vi "Code 0.0.3.vi"() -> ()   [LabVIEW 2017]
uses:
  <vilib>/Instr/_visa.llb/VISA Open Access Mode.ctl
  <vilib>/Instr/_visa.llb/Select Event Type.ctl
  <vilib>/Utility/config.llb/Read Key (String).vi
  <vilib>/Utility/config.llb/Write Key (String).vi
  <vilib>/Instr/_visa.llb/VISA Configure Serial Port (Instr).vi
  <vilib>/Utility/config.llb/NI_LVConfig.lvlib
panel:
  in  "stop 7":bool
  in  "stop 6":bool
  out "Error List":string
  in  "Flash Baud":u32(ring)=115200 caption="Flash Baudrate" items=["4800"=4800, "9600"=9600, "19200"=19200, "38400"=38400, "57600"=57600, "115200"=115200, "230400"=230400, "460800"=460800, "921600"=921600]
  in  "cmd Baud":u32(ring)=230400 items=["4800"=4800, "9600"=9600, "19200"=19200, "38400"=38400, "57600"=57600, "115200"=115200, "230400"=230400, "460800"=460800, "921600"=921600]
  in  "COM Port":refnum<visa-resource-name>="COM4"
  in  "Next Button":bool
  in  "File Path Control":path
  out "COM Port":bool
  out "CheckSumArray":u16[][](array[numeric]) format="%.0x"
  out "CheckSum DataB":u16 format="%.0x"
  out "CheckSum Data":u16 format="%.0x"
  out "Array 3":u16[][](array[numeric]) format="%.0x"
  out "Num of Data packet":i32
  out "Size of Text File":i32
  out "Full Text File":u8[](array[numeric]) format="%.0x"
  out "All bytes in file in HEX U8":u8[](array[numeric]) format="%02x"
  out "sumHeader":u16 format="%.0x"
  out "error out":errorcluster
  # "Ver 1.0.5"
  # "© Redler Technologies. All Rights Reserved"
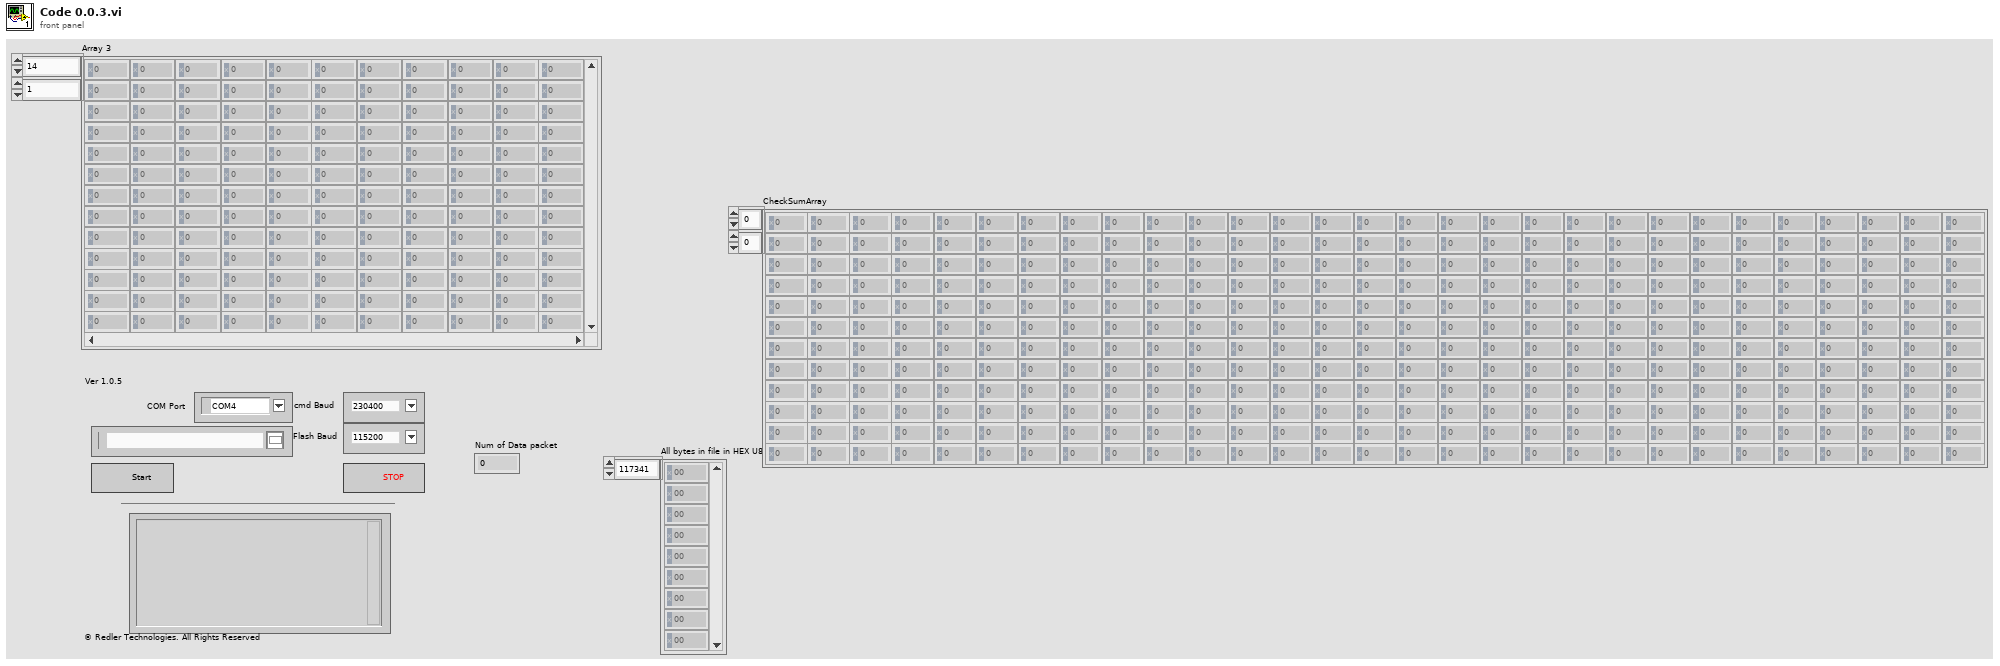
[diagram p1: front panel]
types:
  T1 = typedef "NI_LVConfig.lvlib/Config Data RefNum.ctl" = refnum<k1>
  T2 = typedef "VISA Open Access Mode.ctl" = u32
  T3 = typedef "Select Event Type.ctl" = u32
  T4 = enum16{"open", "replace", "create", "open or create", "replace or create", "replace or create with confirmation"}
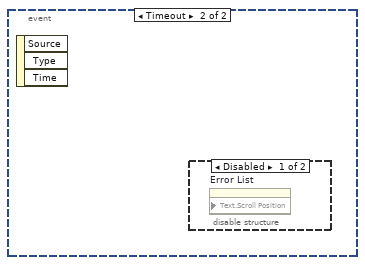
[diagram p3: hidden frame]
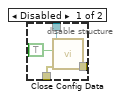
[diagram p5: hidden frame]
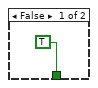
[diagram p6: hidden frame]
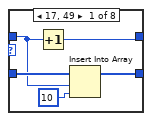
[diagram p7: hidden frame]
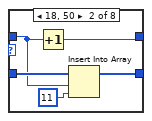
[diagram p8: hidden frame]
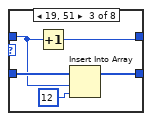
[diagram p9: hidden frame]
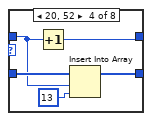
[diagram p10: hidden frame]
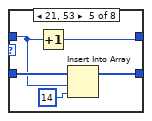
[diagram p11: hidden frame]
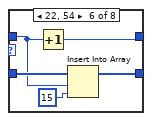
[diagram p12: hidden frame]
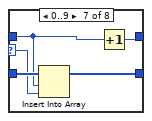
[diagram p13: hidden frame]
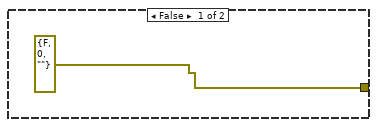
[diagram p15: hidden frame]
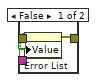
[diagram p16: hidden frame]
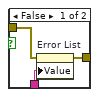
[diagram p18: hidden frame]
diagram:
  w8 = u32 230400 items=["4800"=4800, "9600"=9600, "19200"=19200, "38400"=38400, "57600"=57600, "115200"=115200, "230400"=230400, "460800"=460800, "921600"=921600] ("cmd Baud")
  w9 = u32 230400 items=["4800"=4800, "9600"=9600, "19200"=19200, "38400"=38400, "57600"=57600, "115200"=115200, "230400"=230400, "460800"=460800, "921600"=921600] ("Flash Baud")
  w18 = u32 230400 ("default (0 I32)")
  w3 = "Firmware Path" ("key")
  w4 = "Rayon" ("section")
  n1 = control-ref of="This VI"() -> (w40:refnum<vi>)
  n2 = invoke class="VI" method="Default Vals.Reinit All"(reference=w40, error in=errorcluster {"status"=FALSE, "code"=0, "source"=""} ("error in (no error)")) -> (error out=w7:errorcluster)  [unwired: 1 in, 2 out]
  n3 = property on="Flash Baud" class="Ring (strict)"(error in=w7, "Value"=w9) -> (error out=w10:errorcluster)  [unwired: 1 in, 1 out]
  n4 = property on="cmd Baud" class="Ring (strict)"(error in=w10, "Value"=w8) -> (error out=w6:errorcluster)  [unwired: 1 in, 1 out]
  n5 = call <vilib>:"Application Directory.vi"() -> ("Application Directory"=w38:path)
  n6 = Build Path(base path=w38, name or relative path="data\\RayonSerialProgramerConfigurationFile.ini") -> (appended path=w29:path)
  n7 = call <vilib>:"Open Config Data.vi"("error in (no error)"=w6, "create file if necessary (T)"=FALSE, "configuration file path"=w29) -> ("error out"=w34:errorcluster, "refnum"=w35:T1)  [unwired: 7 out]
  n8 = call-poly <vilib>:"Read Key.vi"("section"=w4, "error in (no error)"=w34, "key"=w3, "refnum"=w35) -> ("error out"=w1:errorcluster, "value"=w33:string, "refnum out"=w5:T1)  [unwired: 2 in, 3 out]
  n9 = String To Path(string=w33) -> (path=w32:path)
  n10 = property on="File Path Control" class="Path"(error in=w1, "Value"=w32) -> (error out=w2:errorcluster)  [unwired: 1 in, 1 out]
  n11 = call-poly <vilib>:"Read Key.vi"("section"=w4, "error in (no error)"=w2, "key"="COM", "refnum"=w5) -> ("error out"=w22:errorcluster, "value"=w14:string, "refnum out"=w27:T1)  [unwired: 2 in, 3 out]
  n12 = Type Cast(type=refnum<visa-resource-name> "COM1" ("UUT COM Port 2"), x=w14) -> (*(type *) &x=w13:refnum<visa-resource-name>)
  n13 = property on="COM Port" class="VISAName"("Value"=w13) -> ()  [unwired: 2 in, 2 out]
  n14 = call-poly <vilib>:"Read Key.vi"("section"=w4, "error in (no error)"=w22, "key"="Flash Baud", "refnum"=w27) -> ("error out"=w21:errorcluster, "value"=w20:string, "refnum out"=w28:T1)  [unwired: 2 in, 3 out]
  n15 = Decimal String To Number(string=w20, default (0L)=w18) -> (number=w16:u32)  [unwired: 1 in, 1 out]
  n16 = property on="Flash Baud" class="Ring (strict)"("Value"=w16) -> ()  [unwired: 2 in, 2 out]
  n17 = call-poly <vilib>:"Read Key.vi"("section"=w4, "error in (no error)"=w21, "key"="Boot Baud", "refnum"=w28) -> ("error out"=w11:errorcluster, "value"=w19:string, "refnum out"=w26:T1)  [unwired: 2 in, 3 out]
  n18 = Decimal String To Number(string=w19, default (0L)=w18) -> (number=w17:u32)  [unwired: 1 in, 1 out]
  n19 = property on="cmd Baud" class="Ring (strict)"("Value"=w17) -> ()  [unwired: 2 in, 2 out]
  n20 = call <vilib>:"Close Config Data.vi"("error in (no error)"=w11, "refnum"=w26) -> ("error out"=w12:errorcluster)  [unwired: 1 in, 8 out]
  n21 = while {
    tunnel: w12 -> [w45]
    tunnel: w4 -> [w107]
    tunnel: w3 -> [w106]
    tunnel: [w108] -> w31
    tunnel: w29 -> [w105]
    stop <- FALSE stop-if-true
    w96 = FALSE ("Next Button")
    w117 = T2 0 items=["VISA Defaults"=0, "Exclusive Lock"=1, "Load Configured Settings"=4] ("Access Mode")
    # "Convert from U8 to U16 to build a word (Header)"
    # "build U8 HEX values"
    # "Convert from U8 to U16 to build a word (Data)"
    # "Convert ASCII string to HEX values"
    n22 = property on="File Path Control" class="Path"(error in=w45, "PTooLngToFt"=enum32{"Abbreviate Path", "Clip Path"}."Abbreviate Path" ("Path Too Long To Fit")) -> ()  [unwired: 1 in, 2 out]
    n23 = property on="stop 6" class="Bool (strict)"(error in=w45, "Value"=FALSE ("stop 6")) -> (error out=w54:errorcluster)  [unwired: 1 in, 1 out]
    n24 = while {
      tunnel: ["COM Port"] -> w43
      tunnel: ["Flash Baud"] -> w119
      tunnel: ["cmd Baud"] -> w118
      tunnel: ["File Path Control"] -> w57
      tunnel: w107 -> [w1024]
      tunnel: w54 -> [w1020]
      tunnel: w106 -> [w1022]
      tunnel: w105 -> [w1018]
      tunnel: [w1010] -> w44
      stop <- w1021 stop-if-true
      n25 = call <vilib>:"Open Config Data.vi"("error in (no error)"=w1020, "create file if necessary (T)"=FALSE, "configuration file path"=w1018) -> ("error out"=w1019:errorcluster, "refnum"=w1016:T1)  [unwired: 7 out]
      n26 = Path To String(path="File Path Control") -> (string=w1023:string)
      n27 = call <vilib>:"Is Path and Not Empty.vi"("path"="File Path Control") -> ("Is Path and Not Empty?"=w1027:bool)  [unwired: 4 in]
      n28 = Not(x=w1027) -> (.not. x?=w1025:bool)
      n29 = And(x=w1025, y="Next Button") -> (x .and. y?=w1026:bool)
      n30 = case shown="False" w1026 {
        tunnel: w1024 -> [w1036 _]
        tunnel: w1019 -> [w1053 w1054]
        tunnel: w1023 -> [w1052 _]
        tunnel: w1022 -> [w1051 _]
        tunnel: w1016 -> [w1050 _]
        tunnel: [w1049 w1055] -> w1010
        tunnel: "COM Port" -> [w1033 _]
        tunnel: "Flash Baud" -> [w1030 _]
        tunnel: "cmd Baud" -> [w1032 _]
        frame False {
          n31 = call-poly <vilib>:"Write Key.vi"("section"=w1036, "error in (no error)"=w1053, "value"=w1052, "key"=w1051, "refnum"=w1050) -> ("error out"=w1043:errorcluster, "refnum out"=w1039:T1)  [unwired: 1 in, 4 out]
          n32 = Type Cast(type="", x=w1033) -> (*(type *) &x=w1031:string)
          n33 = call-poly <vilib>:"Write Key.vi"("section"=w1036, "error in (no error)"=w1043, "value"=w1031, "key"="COM", "refnum"=w1039) -> ("error out"=w1042:errorcluster, "refnum out"=w1038:T1)  [unwired: 1 in, 4 out]
          n34 = Number To Decimal String(number=w1030) -> (decimal integer string=w1048:string)  [unwired: 1 in]
          n35 = call-poly <vilib>:"Write Key.vi"("section"=w1036, "error in (no error)"=w1042, "value"=w1048, "key"="Flash Baud", "refnum"=w1038) -> ("error out"=w1041:errorcluster, "refnum out"=w1037:T1)  [unwired: 1 in, 4 out]
          n36 = Number To Decimal String(number=w1032) -> (decimal integer string=w1045:string)  [unwired: 1 in]
          n37 = call-poly <vilib>:"Write Key.vi"("section"=w1036, "error in (no error)"=w1041, "value"=w1045, "key"="Boot Baud", "refnum"=w1037) -> ("error out"=w1040:errorcluster, "refnum out"=w1035:T1)  [unwired: 1 in, 4 out]
          n38 = call <vilib>:"Close Config Data.vi"("error in (no error)"=w1040, "refnum"=w1035) -> ("error out"=w1049:errorcluster)  [unwired: 1 in, 8 out]
        }
        frame True {
          n39 = One Button Dialog(message="Please select a valid path !") -> ()  [unwired: 1 in, 1 out]
          n40 = property on="Next Button" class="Bool (strict)"(error in=w1054, "Value"=FALSE ("Next Button")) -> (error out=w1055:errorcluster)  [unwired: 1 in, 1 out]
        }
      }
      n41 = property on="Next Button" class="Bool (strict)"("Blinking"="Next Button") -> ()  [unwired: 2 in, 2 out]
      n42 = And(x="Next Button", y=w1027) -> (x .and. y?=w1028:bool)
      n43 = Or(x=w1028, y=FALSE) -> (x .or. y?=w1021:bool)
    }
    n44 = Open/Create/Replace File(file path (use dialog)=w57) -> (refnum out=w61:refnum<file>, error out=w60:errorcluster)  [unwired: 5 in, 1 out]
    n45 = Read from Text File(file (use dialog)=w61, error in=w60) -> (text=w63:string)  [unwired: 2 in, 3 out]
    n46 = String To Byte Array(string=w63) -> (unsigned byte array=w62:u8[])
    n47 = for {
      tunnel: w62 -> [w189] mode=indexing
      shift-right: [w185] -> w66
      shift-left: u8[] [] -> [w186]
      shift-right: [w184] -> _
      shift-left: 0 ("y") -> [w183]
      n48 = Subtract(x=w189, y=u8 48) -> (x-y=w187:u8)
      n49 = case shown="240, Default" w187 {
        selector: w187 -> [_ _ _ _ _ _ w223 _]
        tunnel: [w192 w197 w203 w207 w212 w217 w222 w226] -> w185
        tunnel: w186 -> [w194 w198 w204 w209 w214 w219 w224 w226]
        tunnel: [w190 w195 w200 w205 w210 w215 w220 w225] -> w184
        tunnel: w183 -> [w191 w196 w201 w206 w211 w216 w221 w225]
        frame 17, 49 {
          n50 = Increment(x=w191) -> (x+1=w190:i32)
          n51 = Insert Into Array(array=w194, index=w191, new element=u8 10) -> (w192:u8[])
        }
        frame 18, 50 {
          n52 = Increment(x=w196) -> (x+1=w195:i32)
          n53 = Insert Into Array(array=w198, index=w196, new element=u8 11) -> (w197:u8[])
        }
        frame 19, 51 {
          n54 = Increment(x=w201) -> (x+1=w200:i32)
          n55 = Insert Into Array(array=w204, index=w201, new element=u8 12) -> (w203:u8[])
        }
        frame 20, 52 {
          n56 = Increment(x=w206) -> (x+1=w205:i32)
          n57 = Insert Into Array(array=w209, index=w206, new element=u8 13) -> (w207:u8[])
        }
        frame 21, 53 {
          n58 = Increment(x=w211) -> (x+1=w210:i32)
          n59 = Insert Into Array(array=w214, index=w211, new element=u8 14) -> (w212:u8[])
        }
        frame 22, 54 {
          n60 = Increment(x=w216) -> (x+1=w215:i32)
          n61 = Insert Into Array(array=w219, index=w216, new element=u8 15) -> (w217:u8[])
        }
        frame 0..9 {
          n62 = Insert Into Array(array=w224, index=w221, new element=w223) -> (w222:u8[])
          n63 = Increment(x=w221) -> (x+1=w220:i32)
        }
        frame 240, Default {
        }
      }
    }
    n64 = Array Size(array=w66) -> (size(s)=w67:i32)
    n65 = Divide(x=w67, y=2) -> (x/y=w69:dbl)
    n66 = To Long Integer(number=w69) -> (32bit integer=w70:i32)
    n67 = for {
      N: w70 -> [_]
      tunnel: w66 -> [w182]
      tunnel: [w168] -> w71 mode=indexing
      i -> [w181]
      n68 = Multiply(x=2, y=w181) -> (x*y=w179:i32)
      n69 = Increment(x=w179) -> (x+1=w178:i32)
      n70 = Index Array(array=w182, index #1=w179, index #2=w178) -> (element #1=w171:u8, element #2=w170:u8)
      n71 = Format Into String(w171) -> (resulting string=w172:string)  [unwired: 3 in, 1 out]
      n72 = Format Into String(w170) -> (resulting string=w177:string)  [unwired: 3 in, 1 out]
      n73 = Decimal String To Number(string=w172) -> (number=w173:i32)  [unwired: 2 in, 1 out]
      n74 = Decimal String To Number(string=w177) -> (number=w176:i32)  [unwired: 2 in, 1 out]
      n75 = Multiply(x=w173, y=16) -> (x*y=w175:i32)
      n76 = Add(x=w175, y=w176) -> (x+y=w169:i32)
      n77 = To Unsigned Byte Integer(number=w169) -> (unsigned 8bit integer=w168:u8)
    }
    n78 = Delete From Array(array=w71, length=22, index=0) -> (deleted portion=w82:u8[], array with subset deleted=w59:u8[])
    "All bytes in file in HEX U8" <- w59
    n79 = Array Size(array=w59) -> (size(s)=w76:i32)
    n80 = Array Size(array=w82) -> (size(s)=w77:i32)
    n81 = Divide(x=w76, y=2) -> (x/y=w74:dbl)
    n82 = Divide(x=w77, y=2) -> (x/y=w79:dbl)
    n83 = To Long Integer(number=w74) -> (32bit integer=w81:i32)
    n84 = To Long Integer(number=w79) -> (32bit integer=w80:i32)
    n85 = VISA Flush I/O Buffer(VISA resource name=w43, error in (no error)=w44) -> (VISA resource name out=w41:refnum<visa-resource-name>, error out=w42:errorcluster)  [unwired: 1 in]
    n86 = flat-sequence {
      tunnel: [w137] -> w52
      tunnel: " Openning COM Port..." -> [w136]
      tunnel: w48 -> [_]
      frame #0 {
        n87 = Format Date/Time String(time format string (%c)="%H:%M:%S") -> (date/time string=w135:string)  [unwired: 2 in]
        n88 = Concatenate Strings(w135, w136) -> (w137:string)
      }
    }
    n89 = for {
      N: w81 -> [_]
      tunnel: w59 -> [w164]
      tunnel: [w160] -> w87 mode=indexing
      i -> [w163]
      n90 = Multiply(x=2, y=w163) -> (x*y=w166:i32)
      n91 = Increment(x=w166) -> (x+1=w167:i32)
      n92 = Index Array(array=w164, index #1=w166, index #2=w167) -> (element #1=w162:u8, element #2=w161:u8)
      n93 = Join Numbers(hi=w162, lo=w161) -> ((hi.lo)=w160:u16)
    }
    n94 = for {
      N: w80 -> [_]
      tunnel: w82 -> [w156]
      tunnel: [w152] -> w58 mode=indexing
      i -> [w155]
      n95 = Multiply(x=2, y=w155) -> (x*y=w158:i32)
      n96 = Increment(x=w158) -> (x+1=w159:i32)
      n97 = Index Array(array=w156, index #1=w158, index #2=w159) -> (element #1=w154:u8, element #2=w153:u8)
      n98 = Join Numbers(hi=w154, lo=w153) -> ((hi.lo)=w152:u16)
    }
    n99 = call <vilib>:"Clear Errors.vi"("error in (no error)"=w42) -> ("error out"=w104:errorcluster)  [unwired: 5 in, 1 out]
    n100 = property on="Error List" class="Str"(error in=w104, "Value"="") -> (error out=w48:errorcluster)  [unwired: 1 in, 1 out]
    n101 = Concatenate Strings("\r\n", w52) -> (w112:string)
    n102 = flat-sequence {
      tunnel: [w123] -> w50
      tunnel: [w121] -> w49
      tunnel: w47 -> [_]
      frame #0 {
        n103 = Format Date/Time String(time format string (%c)="%H:%M:%S") -> (date/time string=w128:string)  [unwired: 2 in]
        n104 = Format Date/Time String(time format string (%c)="%H:%M:%S") -> (date/time string=w131:string)  [unwired: 2 in]
        n105 = Format Date/Time String(time format string (%c)="%H:%M:%S") -> (date/time string=w133:string)  [unwired: 2 in]
        n106 = Concatenate Strings(w128, " Openning COM Port success !") -> (w121:string)
        n107 = Concatenate Strings(w131, " Openning COM Port failed !") -> (w124:string)
        n108 = Concatenate Strings(w133, " Check COM adaptor." ("string"), "\r\n") -> (w125:string)
        n109 = Concatenate Strings(w125, w124) -> (w123:string)
      }
    }
    n110 = property on="Error List" class="Str"(error in=w48, "Value"=w112) -> (error out=w111:errorcluster)  [unwired: 1 in, 1 out]
    n111 = Index Array(array=w58, index=0) -> (element=w89:u16)
    n112 = Not Equal?(x=w89, y=u16 43528) -> (x != y?=w91:bool)
    n113 = VISA Open(access mode=w117, error in (no error)=w111, VISA resource name=w41) -> (VISA resource name=w116:refnum<visa-resource-name>, error out=w115:errorcluster)  [unwired: 2 in]
    n114 = case shown="True" w91 {
      tunnel: [TRUE FALSE] -> w55
      frame False {
      }
      frame True {
        n115 = One Button Dialog(message="Wrong file format.\nReplace file. ") -> ()  [unwired: 1 in, 1 out]
      }
    }
    n116 = VISA Clear(VISA resource name=w116, error in (no error)=w115) -> (VISA resource name out=w53:refnum<visa-resource-name>, error out=w47:errorcluster)
    n117 = Unbundle By Name(w47) -> ("status"=w92:bool)
    n118 = call <vilib>:"Clear Errors.vi"("error in (no error)"=w47) -> ("error out"=w99:errorcluster)  [unwired: 5 in, 1 out]
    n119 = Select(t=w50, s=w92, f=w49) -> (s? t:f=w102:string)
    n120 = property on="Error List" class="Str"(error in=w99) -> (error out=w94:errorcluster, "Value"=w110:string)  [unwired: 1 in, 1 out]
    n121 = case shown="True" w92 {
      tunnel: w94 -> [w227 w231]
      tunnel: [w227 w230] -> w93
      tunnel: w53 -> [_ w229]
      frame False {
      }
      frame True {
        n122 = call "Time Delay"("error in (no error)"=w231) -> ("error out"=w230:errorcluster)  [unwired: 10 in]
        n123 = VISA Close(VISA resource name=w229, error in (no error)=w230) -> (error out=w228:errorcluster)
        n124 = call <vilib>:"Clear Errors.vi"("error in (no error)"=w228) -> ()  [unwired: 5 in, 2 out]
      }
    }
    n125 = Not(x=w92) -> (.not. x?=w100:bool)
    "COM Port" <- w100
    n126 = Concatenate Strings(w102, w110) -> (w114:string)
    n127 = property on="Error List" class="Str"(error in=w93, "Value"=w114) -> (error out=w113:errorcluster)  [unwired: 1 in, 1 out]
    n128 = And(x=w55, y=w100) -> (x .and. y?=w56:bool)
    n129 = case shown="True" w56 {
      tunnel: w119 -> [_ w321]
      tunnel: w118 -> [_ w320]
      tunnel: w113 -> [_ w311]
      tunnel: w53 -> [_ w310]
      tunnel: w100 -> [_ w308]
      tunnel: [errorcluster {"status"=FALSE, "code"=0, "source"=""} ("error out") w273] -> w109
      tunnel: w59 -> [_ w276]
      tunnel: w58 -> [_ w275]
      frame False {
      }
      frame True {
        w326 = u16 0 items=["None", "LastBit", "TermChar", "Break"] ("Serial Settings:Serial End Mode for Writes")
        w329 = u16 0 items=["None", "XON/XOFF", "RTS/CTS", "XON/XOFF & RTS/CTS", "DTR/DSR", "XON/XOFF & DTR/DSR"] ("flow control (0:none)")
        w330 = u16 10 items=["1.0"=10, "1.5"=15, "2.0"=20] ("stop bits (10: 1 bit)")
        (unwired) "uRayonM1_1.05.01_HW2.txt" ("name or relative path")
        (unwired) u16[] [1536, 15872, 128, 15912, 0, 37503, 63861, 36326, 15872] ("Array 4")
        # "Receive header checksum from the UUT"
        # "- U16 array to be send in string\n- Perform the header checksum"
        n130 = case shown="True" w308 {
          tunnel: w311 -> [w524 w534]
          tunnel: w310 -> [w523 w540]
          tunnel: [w523 w536] -> w309
          tunnel: [w524 w537] -> w294
          tunnel: [0 ("D Int out") w539] -> w301
          tunnel: [FALSE w538] -> w274
          tunnel: [TRUE ("Value") w525] -> w236
          frame False {
          }
          frame True {
            w530 = "\r\n"
            w551 = u16 0 items=["None", "XON/XOFF", "RTS/CTS", "XON/XOFF & RTS/CTS", "DTR/DSR", "XON/XOFF & DTR/DSR"] ("flow control (0:none)")
            w550 = u16 10 items=["1.0"=10, "1.5"=15, "2.0"=20] ("stop bits (10: 1 bit)")
            w552 = T3 1073684533 items=["Service Request"=1073684491, "Trigger"=3221168138, "Clear"=1073684493, "VXI Signal"=1073684512, "VXI/VME Interrupt"=3221168161, "VXI/VME Sysfail"=1073684509, "VXI/VME Sysreset"=1073684510, "GPIB CIC"=1073684498, "GPIB Talk"=1073684499, "GPIB Listen"=1073684500, "PXI Interrupt"=1073684514, "Serial Break"=1073684515, "Serial TermChar"=1073684516, "Serial CTS"=1073684521, "Serial DSR"=1073684522, "Serial DCD"=1073684524, "Serial RI"=1073684526, "Serial Character"=1073684533, "USB Interrupt"=1073684535, "All Enabled"=1073709055] ("Event Type")
            n131 = property on="Error List" class="Str"(error in=w534) -> (error out=w533:errorcluster, "Value"=w531:string)  [unwired: 1 in, 1 out]
            n132 = Format Date/Time String(time format string (%c)="%H:%M:%S") -> (date/time string=w528:string)  [unwired: 2 in]
            n133 = Concatenate Strings(w528, " Getting Driver version...") -> (w526:string)
            n134 = Concatenate Strings(w526, w530, w531, w530) -> (w535:string)
            n135 = property on="Error List" class="Str"(error in=w533, "Value"=w535) -> (error out=w532:errorcluster)  [unwired: 1 in, 1 out]
            n136 = call-poly "VISA Configure Serial Port"("VISA resource name"=w540, "timeout (10sec)"=u32 200, "Enable Termination\nChar (T)"=FALSE ("Enable Termination\nChar (T)"), "baud rate (9600)"=u32 230400, "data bits (8)"=u16 8, "parity (0:none)"=enum16{"None", "Odd", "Even", "Mark", "Space"}."None", "error in (no error)"=w532, "stop bits (10: 1 bit)"=w550, "flow control (0:none)"=w551) -> ("VISA resource name out"=w544:refnum<visa-resource-name>, "error out"=w545:errorcluster)  [unwired: 5 in]
            n137 = VISA Enable Event(8:w545, 10:w552, 11:w544) -> (0:w542:errorcluster, 3:w543:refnum<visa-resource-name>)  [unwired: 1 in]
            n138 = Byte Array To String(unsigned byte array=u8[] [73, 93, 62, 192, 16, 48, 0] ("output array")) -> (string=w556:string)
            n139 = VISA Write(VISA resource name=w543, write buffer=w556, error in (no error)=w542) -> (VISA resource name out=w558:refnum<visa-resource-name>, error out=w555:errorcluster)  [unwired: 1 out]
            n140 = flat-sequence {
              tunnel: w555 -> [w560]
              tunnel: [w560] -> w554
              tunnel: [w559] -> w553
              frame #0 {
                n141 = call <vilib>:"High Resolution Relative Seconds.vi"() -> ("relative seconds"=w559:dbl)
              }
            }
            n142 = while {
              tunnel: w554 -> [w578]
              tunnel: [w575] -> w537
              tunnel: w558 -> [w577]
              tunnel: [w576] -> w536
              tunnel: w553 -> [w568]
              tunnel: [w563] -> w539
              tunnel: [w562] -> w538
              tunnel: [w561] -> w525
              stop <- w565 stop-if-true
              n143 = call <vilib>:"High Resolution Relative Seconds.vi"() -> ("relative seconds"=w569:dbl)
              n144 = VISA Read(VISA resource name=w577, byte count=u32 11, error in (no error)=w578) -> (VISA resource name out=w576:refnum<visa-resource-name>, read buffer=w573:string, return count=w570:u32, error out=w575:errorcluster)
              n145 = Subtract(x=w569, y=w568) -> (x-y=w566:dbl)
              n146 = String To Byte Array(string=w573) -> (unsigned byte array=w572:u8[])
              n147 = Not Equal To 0?(x=w570) -> (x != 0?=w562:bool)
              n148 = Greater Or Equal?(x=w566, y=3.0) -> (x >= y?=w564:bool)
              n149 = call "Data_Convert.vi"("Data Type"=u8 0, "Array"=w572) -> ("D Int out"=w563:i32)  [unwired: 2 out]
              n150 = property on="stop 6" class="Bool (strict)"() -> ("Value"=w561:bool)  [unwired: 2 in, 2 out]
              n151 = Compound Arithmetic op=OR(w561, w562, w564) -> (w565:bool)
            }
          }
        }
        n152 = flat-sequence {
          tunnel: [w396] -> w254
          tunnel: [w392] -> w253
          tunnel: [w390] -> w252
          tunnel: [w388] -> w251
          tunnel: [" Sending autobaud operation..." ("string")] -> w250
          tunnel: [" Getting Driver version failed !" ("f")] -> w249
          tunnel: ["\r\n"] -> w248
          tunnel: w244 -> [_]
          frame #0 {
            n153 = Format Date/Time String(time format string (%c)="%H:%M:%S") -> (date/time string=w398:string)  [unwired: 2 in]
            n154 = Format Date/Time String(time format string (%c)="%H:%M:%S") -> (date/time string=w394:string)  [unwired: 2 in]
            n155 = Format Date/Time String(time format string (%c)="%H:%M:%S") -> (date/time string=w388:string)  [unwired: 2 in]
            n156 = Format Date/Time String(time format string (%c)="%H:%M:%S") -> (date/time string=w390:string)  [unwired: 2 in]
            n157 = Concatenate Strings(w398, " Driver Version: " ("string")) -> (w396:string)
            n158 = Concatenate Strings(w394, " Sending autobaud operation...") -> (w392:string)
          }
        }
        n159 = Concatenate Strings(w251, w249) -> (w246:string)
        n160 = Concatenate Strings(w252, w250, w248) -> (w247:string)
        n161 = call <vilib>:"Clear Errors.vi"("error in (no error)"=w294) -> ("error out"=w284:errorcluster)  [unwired: 5 in, 1 out]
        n162 = Format Into String(w301) -> (resulting string=w255:string)  [unwired: 3 in, 1 out]
        n163 = Concatenate Strings(w247, w246) -> (w245:string)
        n164 = property on="Error List" class="Str"(error in=w284) -> (error out=w244:errorcluster, "Value"=w257:string)  [unwired: 1 in, 1 out]
        n165 = Concatenate Strings(w253, "\r\n", w254, w255) -> (w282:string)
        n166 = Select(t=w282, s=w274, f=w245) -> (s? t:f=w270:string)
        n167 = Concatenate Strings(w270, "\r\n", w257) -> (w302:string)
        n168 = case shown="False" w236 {
          tunnel: w302 -> [w363 _]
          tunnel: [w362 w364] -> w300
          tunnel: w244 -> [w361 w364]
          frame False {
            n169 = property on="Error List" class="Str"(error in=w361, "Value"=w363) -> (error out=w362:errorcluster)  [unwired: 1 in, 1 out]
          }
          frame True {
          }
        }
        n170 = call <vilib>:"Clear Errors.vi"("error in (no error)"=w300) -> ("error out"=w289:errorcluster)  [unwired: 5 in, 1 out]
        n171 = call-poly "VISA Configure Serial Port"("VISA resource name"=w309, "timeout (10sec)"=u32 200, "termination char\n(0xA = '\\n' = LF)"=u8 10 ("termination char\n(0xA = '\\n' = LF)"), "Enable Termination\nChar (T)"=FALSE ("Enable Termination\nChar (T)"), "baud rate (9600)"=w320, "data bits (8)"=u16 8, "parity (0:none)"=enum16{"None", "Odd", "Even", "Mark", "Space"}."None", "error in (no error)"=w289, "stop bits (10: 1 bit)"=w330, "flow control (0:none)"=w329) -> ("VISA resource name out"=w327:refnum<visa-resource-name>, "error out"=w328:errorcluster)  [unwired: 4 in]
        n172 = property class="Instr"(reference=w327, error in=w328, "Serial Settings:End Mode for Writes"=w326, "Message Based Settings:Send End Enable"=FALSE) -> (reference out=w323:refnum<visa-resource-name>, error out=w319:errorcluster)
        n173 = flat-sequence {
          tunnel: w319 -> [w580]
          tunnel: [w580] -> w318
          tunnel: [w579] -> w317
          frame #0 {
            n174 = call <vilib>:"High Resolution Relative Seconds.vi"() -> ("relative seconds"=w579:dbl)
          }
        }
        n175 = while {
          tunnel: [w587] -> w344
          tunnel: [w588] -> w343
          tunnel: w321 -> [w601]
          tunnel: w317 -> [w592]
          tunnel: w318 -> [w612]
          tunnel: [w614] -> w293
          tunnel: w323 -> [w613]
          tunnel: [w615] -> w342
          tunnel: [w589] -> _
          tunnel: [w583] -> w281
          tunnel: w274 -> [_]
          tunnel: [w581] -> w235
          i -> [w606]
          stop <- w609 stop-if-true
          w594 = u16 0 items=["None", "XON/XOFF", "RTS/CTS", "XON/XOFF & RTS/CTS", "DTR/DSR", "XON/XOFF & DTR/DSR"] ("flow control (0:none)")
          w595 = u16 10 items=["1.0"=10, "1.5"=15, "2.0"=20] ("stop bits (10: 1 bit)")
          w588 = "A" ("write buffer")
          # "Send cmd for bootloader enable"
          # "Send 'A' for autobaud"
          n176 = case shown="True" TRUE {
            tunnel: w613 -> [w633 w640]
            tunnel: w612 -> [w632 w639]
            tunnel: [w633 w638] -> w602
            tunnel: [w632 w634] -> w603
            tunnel: u8[] [73, 93, 65, 0, 0, 1, 0, 0, 0, 80, 248] ("output array") -> [_ w636]
            frame False {
            }
            frame True {
              n177 = Byte Array To String(unsigned byte array=w636) -> (string=w635:string)
              n178 = VISA Write(VISA resource name=w640, write buffer=w635, error in (no error)=w639) -> (VISA resource name out=w638:refnum<visa-resource-name>, error out=w637:errorcluster)  [unwired: 1 out]
              n179 = call "Time Delay2"("error in (no error)"=w637) -> ("error out"=w634:errorcluster)  [unwired: 10 in]
            }
          }
          n180 = call-poly "VISA Configure Serial Port"("VISA resource name"=w602, "timeout (10sec)"=u32 200, "termination char\n(0xA = '\\n' = LF)"=u8 10 ("termination char\n(0xA = '\\n' = LF)"), "Enable Termination\nChar (T)"=FALSE ("Enable Termination\nChar (T)"), "baud rate (9600)"=w601, "data bits (8)"=u16 8, "parity (0:none)"=enum16{"None", "Odd", "Even", "Mark", "Space"}."None", "error in (no error)"=w603, "stop bits (10: 1 bit)"=w595, "flow control (0:none)"=w594) -> ("VISA resource name out"=w604:refnum<visa-resource-name>, "error out"=w605:errorcluster)  [unwired: 4 in]
          n181 = call <vilib>:"High Resolution Relative Seconds.vi"() -> ("relative seconds"=w593:dbl)
          n182 = VISA Write(VISA resource name=w604, write buffer=w588, error in (no error)=w605) -> (VISA resource name out=w610:refnum<visa-resource-name>, error out=w586:errorcluster)  [unwired: 1 out]
          n183 = flat-sequence {
            tunnel: w586 -> [w617]
            tunnel: [w617] -> w585
            tunnel: [w616] -> w584
            frame #0 {
              n184 = call <vilib>:"High Resolution Relative Seconds.vi"() -> ("relative seconds"=w616:dbl)
            }
          }
          n185 = Subtract(x=w593, y=w592) -> (x-y=w591:dbl)
          n186 = while {
            tunnel: [w627] -> w587
            tunnel: w584 -> [w621]
            tunnel: w585 -> [w628]
            tunnel: [w623] -> w614
            tunnel: w610 -> [w629]
            tunnel: [w631] -> w615
            stop <- w624 stop-if-true
            n187 = call <vilib>:"High Resolution Relative Seconds.vi"() -> ("relative seconds"=w622:dbl)
            n188 = VISA Read(VISA resource name=w629, byte count=u32 1, error in (no error)=w628) -> (VISA resource name out=w631:refnum<visa-resource-name>, read buffer=w627:string, error out=w623:errorcluster)  [unwired: 1 out]
            n189 = Subtract(x=w622, y=w621) -> (x-y=w620:dbl)
            n190 = Greater Or Equal?(x=w620, y=0.2) -> (x >= y?=w619:bool)
            n191 = Equal?(x="A", y=w627) -> (x = y?=w625:bool)
            n192 = Or(x=w625, y=w619) -> (x .or. y?=w624:bool)
          }
          n193 = Greater Or Equal?(x=w591, y=3.0) -> (x >= y?=w589:bool)
          n194 = Equal?(x=w588, y=w587) -> (x = y?=w583:bool)
          n195 = property on="stop 6" class="Bool (strict)"() -> ("Value"=w581:bool)  [unwired: 2 in, 2 out]
          n196 = Equal?(x=5, y=w606) -> (x = y?=w607:bool)
          n197 = Compound Arithmetic op=OR(w583, w607, w581) -> (w609:bool)
        }
        n198 = call <vilib>:"Application Directory.vi"() -> ("Application Directory"=w339:path)
        n199 = Build Path(base path=w339, name or relative path="uRayonM1_1.03.02.txt") -> ()  [unwired: 1 out]
        n200 = flat-sequence {
          tunnel: [w371] -> w243
          tunnel: [w365] -> w242
          tunnel: w241 -> [_]
          frame #0 {
            n201 = Format Date/Time String(time format string (%c)="%H:%M:%S ") -> (date/time string=w380:string)  [unwired: 2 in]
            n202 = Format Date/Time String(time format string (%c)="%H:%M:%S ") -> (date/time string=w379:string)  [unwired: 2 in]
            n203 = Format Date/Time String(time format string (%c)="%H:%M:%S ") -> (date/time string=w378:string)  [unwired: 2 in]
            n204 = Format Date/Time String(time format string (%c)="%H:%M:%S ") -> (date/time string=w377:string)  [unwired: 2 in]
            n205 = Concatenate Strings(w380, "Erase start..." ("string"), "\r\n") -> (w367:string)
            n206 = Concatenate Strings(w379, "Autobaud handshake success !") -> (w366:string)
            n207 = Concatenate Strings(w378, "Try changing baudrate, verify COM adaptor, Power Supply and reset unit.", "\r\n") -> (w373:string)
            n208 = Concatenate Strings(w377, "No response, autobaud handshake failed !" ("string")) -> (w372:string)
            n209 = Concatenate Strings(w367, w366) -> (w365:string)
            n210 = Concatenate Strings(w373, w372) -> (w371:string)
          }
        }
        n211 = Equal?(x=w343, y=w344) -> (x = y?=w316:bool)
        n212 = call <vilib>:"Clear Errors.vi"("error in (no error)"=w293) -> ("error out"=w290:errorcluster)  [unwired: 5 in, 1 out]
        n213 = property on="Error List" class="Str"(error in=w290) -> (error out=w241:errorcluster, "Value"=w259:string)  [unwired: 1 in, 1 out]
        n214 = Select(t=w242, s=w281, f=w243) -> (s? t:f=w269:string)
        n215 = Concatenate Strings(w269, "\r\n", w259) -> (w307:string)
        n216 = case shown="False" w235 {
          tunnel: w307 -> [w359 _]
          tunnel: [w358 w360] -> w306
          tunnel: w241 -> [w357 w360]
          frame False {
            n217 = property on="Error List" class="Str"(error in=w357, "Value"=w359) -> (error out=w358:errorcluster)  [unwired: 1 in, 1 out]
          }
          frame True {
          }
        }
        n218 = flat-sequence {
          tunnel: w306 -> [w991]
          tunnel: [w996] -> w341
          tunnel: [w993] -> w340
          tunnel: w275 -> [w992]
          tunnel: [w991] -> w324
          frame #0 {
            (unwired) u16[] [43528, 0, 0, 0, 0, 0, 0, 0, 0, 15872, 36326]
            n219 = for {
              tunnel: w992 -> [w1009] mode=indexing
              shift-right: [w1004] -> w996
              shift-left: u8[] [] -> [w1003]
              shift-right: [w1001] -> w995
              shift-left: u16 0 -> [w1002]
              i -> [w1008]
              n220 = Split Number(x=w1009) -> (hi(x)=w1000:u8, lo(x)=w999:u8)
              n221 = Build Array(w1000, w999) -> (w1006:u8[])
              n222 = Compound Arithmetic op=ADD(w1002, w1000, w999) -> (w1001:u16)
              n223 = Multiply(x=w1008, y=2) -> (x*y=w1005:i32)
              n224 = Insert Into Array(array=w1003, index=w1005, new element=w1006) -> (w1004:u8[])
            }
            "sumHeader" <- w995
            n225 = Type Cast(type="", x=w995) -> (*(type *) &x=w993:string)
          }
        }
        n226 = And(x=w316, y=TRUE) -> (x .and. y?=w315:bool)
        n227 = case shown="True" w315 {
          tunnel: w324 -> [w934 w940]
          tunnel: w342 -> [w935 w941]
          tunnel: [w934 w953] -> w292
          tunnel: [w935 w952] -> w335
          tunnel: w341 -> [_ w936]
          tunnel: ["0" ("read buffer") w951] -> w338
          tunnel: ["0" ("read buffer") w950] -> w337
          tunnel: [TRUE w942] -> _
          frame False {
          }
          frame True {
            n228 = Byte Array To String(unsigned byte array=w936) -> (string=w937:string)
            n229 = VISA Write(VISA resource name=w941, write buffer=w937, error in (no error)=w940) -> (VISA resource name out=w938:refnum<visa-resource-name>, error out=w939:errorcluster)  [unwired: 1 out]
            n230 = flat-sequence {
              tunnel: w939 -> [w958]
              tunnel: [w958] -> w949
              tunnel: [w957] -> w948
              frame #0 {
                n231 = call <vilib>:"High Resolution Relative Seconds.vi"() -> ("relative seconds"=w957:dbl)
              }
            }
            n232 = while {
              tunnel: w938 -> [w987]
              tunnel: [w988] -> w954
              tunnel: w949 -> [w986]
              tunnel: [w989] -> w947
              tunnel: [w981] -> w950
              tunnel: w948 -> [w977]
              tunnel: [w975] -> w943
              stop <- w983 stop-if-true
              n233 = VISA Read(VISA resource name=w987, byte count=u32 1, error in (no error)=w986) -> (VISA resource name out=w988:refnum<visa-resource-name>, read buffer=w981:string, return count=w982:u32, error out=w989:errorcluster)
              n234 = call <vilib>:"High Resolution Relative Seconds.vi"() -> ("relative seconds"=w978:dbl)
              n235 = Not Equal?(x=w982, y=u32 0) -> (x != y?=w984:bool)
              n236 = Subtract(x=w978, y=w977) -> (x-y=w979:dbl)
              n237 = property on="stop 6" class="Bool (strict)"() -> ("Value"=w976:bool)  [unwired: 2 in, 2 out]
              n238 = Greater Or Equal?(x=w979, y=10.0) -> (x >= y?=w975:bool)
              n239 = Compound Arithmetic op=OR(w984, w976, w975) -> (w983:bool)
              n240 = property on="stop 6" class="Bool (strict)"("Value"=w975) -> ()  [unwired: 2 in, 2 out]
            }
            n241 = flat-sequence {
              tunnel: w947 -> [w955]
              tunnel: [w956] -> w945
              tunnel: [w955] -> w946
              frame #0 {
                n242 = call <vilib>:"High Resolution Relative Seconds.vi"() -> ("relative seconds"=w956:dbl)
              }
            }
            n243 = while {
              tunnel: w954 -> [w973]
              tunnel: [w970] -> w952
              tunnel: w946 -> [w974]
              tunnel: [w971] -> w953
              tunnel: [w965] -> w951
              tunnel: w945 -> [w961]
              tunnel: [w960] -> w944
              stop <- w966 stop-if-true
              n244 = VISA Read(VISA resource name=w973, byte count=u32 1, error in (no error)=w974) -> (VISA resource name out=w970:refnum<visa-resource-name>, read buffer=w965:string, return count=w967:u32, error out=w971:errorcluster)
              n245 = call <vilib>:"High Resolution Relative Seconds.vi"() -> ("relative seconds"=w964:dbl)
              n246 = Not Equal?(x=w967, y=u32 0) -> (x != y?=w969:bool)
              n247 = Subtract(x=w964, y=w961) -> (x-y=w963:dbl)
              n248 = property on="stop 6" class="Bool (strict)"() -> ("Value"=w959:bool)  [unwired: 2 in, 2 out]
              n249 = Greater Or Equal?(x=w963, y=10.0) -> (x >= y?=w960:bool)
              n250 = Compound Arithmetic op=OR(w969, w959, w960) -> (w966:bool)
            }
            n251 = Or(x=w944, y=w943) -> (x .or. y?=w942:bool)
          }
        }
        n252 = call <vilib>:"Clear Errors.vi"("error in (no error)"=w292) -> ("error out"=w283:errorcluster)  [unwired: 5 in, 1 out]
        n253 = property on="Error List" class="Str"(error in=w283) -> (error out=w240:errorcluster, "Value"=w261:string)  [unwired: 1 in, 1 out]
        n254 = Concatenate Strings(w338, w337) -> (w336:string)
        n255 = Equal?(x=w340, y=w336) -> (x = y?=w278:bool)
        n256 = case shown="True" w281 {
          tunnel: w278 -> [_ w446]
          tunnel: ["" w445] -> w268
          tunnel: w240 -> [_ w442]
          frame False {
          }
          frame True {
            n257 = flat-sequence {
              tunnel: [w453] -> w443
              tunnel: [w447] -> w444
              tunnel: w442 -> [_]
              frame #0 {
                n258 = Format Date/Time String(time format string (%c)="%H:%M:%S ") -> (date/time string=w462:string)  [unwired: 2 in]
                n259 = Format Date/Time String(time format string (%c)="%H:%M:%S ") -> (date/time string=w461:string)  [unwired: 2 in]
                n260 = Format Date/Time String(time format string (%c)="%H:%M:%S ") -> (date/time string=w460:string)  [unwired: 2 in]
                n261 = Format Date/Time String(time format string (%c)="%H:%M:%S ") -> (date/time string=w459:string)  [unwired: 2 in]
                n262 = Concatenate Strings(w462, "Program start..." ("string"), "\r\n") -> (w449:string)
                n263 = Concatenate Strings(w461, "Erase success !") -> (w448:string)
                n264 = Concatenate Strings(w460, "Please check COM adaptor, Power Supply and reset unit.", "\r\n") -> (w455:string)
                n265 = Concatenate Strings(w459, "No response, Erase failed !" ("string")) -> (w454:string)
                n266 = Concatenate Strings(w449, w448) -> (w447:string)
                n267 = Concatenate Strings(w455, w454) -> (w453:string)
              }
            }
            n268 = Select(t=w444, s=w446, f=w443) -> (s? t:f=w445:string)
          }
        }
        n269 = Concatenate Strings(w268, "\r\n", w261) -> (w305:string)
        n270 = And(x=w278, y=TRUE) -> (x .and. y?=w313:bool)
        n271 = case shown="True" w235 {
          tunnel: w305 -> [w355 _]
          tunnel: [w354 w356] -> w304
          tunnel: w240 -> [w353 w356]
          frame False {
            n272 = property on="Error List" class="Str"(error in=w353, "Value"=w355) -> (error out=w354:errorcluster)  [unwired: 1 in, 1 out]
          }
          frame True {
          }
        }
        n273 = case shown="True" w313 {
          tunnel: w335 -> [w643 w650]
          tunnel: [w643 w649] -> w299
          tunnel: [w641 w647] -> w280
          tunnel: w276 -> [_ w651]
          tunnel: [FALSE w645] -> w271
          tunnel: w304 -> [w641 w646]
          tunnel: 0.001 ("Delay Time (s)") -> [_ w644]
          frame False {
          }
          frame True {
            n274 = for {
              shift-right: [w677] -> _
              shift-left: w651 -> [w688]
              tunnel: w651 -> [_] mode=indexing
              tunnel: [w670] -> w652 mode=indexing
              tunnel: w650 -> [w669]
              tunnel: [w666] -> w649
              tunnel: [w655] -> _ mode=concatenating
              tunnel: [w664] -> w648 mode=indexing
              shift-right: [w665] -> w647
              shift-left: w646 -> [w658]
              tunnel: [w657] -> w645
              tunnel: [w655] -> _ mode=indexing
              tunnel: w644 -> [w653]
              i -> [w678]
              stop <- w656 stop-if-true
              n275 = Increment(x=w678) -> (x+1=→"Num of Data packet":i32)
              n276 = Index Array(array=w688) -> (element #1=w687:u8, element #2=w686:u8)  [unwired: 2 in]
              n277 = Join Numbers(hi=w686, lo=w687) -> ((hi.lo)=w660:u16)
              n278 = Add(x=w660, y=u32 3) -> (x+y=w684:u32)
              n279 = property on="stop 6" class="Bool (strict)"() -> ("Value"=w654:bool)  [unwired: 2 in, 2 out]
              n280 = Equal?(x=w660, y=u16 0) -> (x = y?=w681:bool)
              n281 = Multiply(x=w684, y=u32 2) -> (x*y=w682:u32)
              n282 = Or(x=w681, y=w654) -> (x .or. y?=w656:bool)
              n283 = To Long Integer(number=w682) -> (32bit integer=w661:i32)
              n284 = Delete From Array(array=w688, length=w661, index=0) -> (deleted portion=w662:u8[], array with subset deleted=w677:u8[])
              n285 = Array Size(array=w662) -> (size(s)=w674:i32)
              n286 = Divide(x=w674, y=2) -> (x/y=w676:dbl)
              n287 = To Long Integer(number=w676) -> (32bit integer=w673:i32)
              n288 = for {
                N: w673 -> [_]
                tunnel: w662 -> [w927]
                tunnel: [w923] -> w670 mode=indexing
                i -> [w926]
                n289 = Multiply(x=2, y=w926) -> (x*y=w929:i32)
                n290 = Increment(x=w929) -> (x+1=w930:i32)
                n291 = Index Array(array=w927, index #1=w929, index #2=w930) -> (element #1=w925:u8, element #2=w924:u8)
                n292 = Join Numbers(hi=w925, lo=w924) -> ((hi.lo)=w923:u16)
              }
              n293 = Array Size(array=w670) -> (size(s)=w672:i32)
              n294 = Equal?(x=w661, y=6) -> (x = y?=w659:bool)
              n295 = Less Or Equal?(x=w672, y=1027) -> (x <= y?=w667:bool)
              n296 = case shown="False" w654 {
                tunnel: w670 -> [w701 _]
                tunnel: w669 -> [w700 w921]
                tunnel: w667 -> [w699 _]
                tunnel: [w697 w921] -> w666
                tunnel: [w696 w920] -> w665
                tunnel: [w695 u16[] []] -> w664
                tunnel: w659 -> [w694 _]
                tunnel: w658 -> [w693 w920]
                tunnel: [w690 TRUE] -> w657
                tunnel: [w691 bool[] []] -> w655
                tunnel: w653 -> [w689 _]
                frame False {
                  n297 = Or(x=w694, y=w699) -> (x .or. y?=w698:bool)
                  n298 = case shown="True" w698 {
                    tunnel: w693 -> [w707 w838]
                    tunnel: w700 -> [w710 w829]
                    tunnel: [w709 w824] -> w696
                    tunnel: [w708 w840] -> w697
                    tunnel: w701 -> [w705 w839]
                    tunnel: [w706 w836] -> w691
                    tunnel: [w704 w834] -> w695
                    tunnel: w694 -> [_ w833]
                    tunnel: [w703 w823] -> w692
                    tunnel: w689 -> [w702 w822]
                    frame False {
                      n299 = while {
                        tunnel: w705 -> [_]
                        tunnel: [w713] -> w706 mode=concatenating
                        shift-right: [w733] -> w708
                        shift-left: w710 -> [w734]
                        shift-right: [w716] -> w709
                        shift-left: w707 -> [w732]
                        shift-right: [w725] -> _
                        shift-left: w705 -> [w731]
                        tunnel: [w724] -> w704 mode=indexing
                        tunnel: [w712] -> w703
                        tunnel: w702 -> [w711]
                        i -> [w723]
                        stop <- w715 stop-if-true
                        n300 = Equal To 0?(x=w723) -> (x = 0?=w722:bool)
                        n301 = Select(t=1027 ("length"), s=w722, f=1024 ("length")) -> (s? t:f=w719:i32)
                        n302 = Delete From Array(array=w731, length=w719, index=0) -> (deleted portion=w726:u16[], array with subset deleted=w725:u16[])
                        n303 = property on="stop 6" class="Bool (strict)"() -> ("Value"=w714:bool)  [unwired: 2 in, 2 out]
                        n304 = Array Size(array=w726) -> (size(s)=w729:i32)
                        n305 = Greater?(x=w729, y=1) -> (0:w727:bool)
                        n306 = Not(x=w727) -> (.not. x?=w717:bool)
                        n307 = Or(x=w717, y=w714) -> (x .or. y?=w715:bool)
                        n308 = case shown="True" w727 {
                          tunnel: w734 -> [w737 w765]
                          tunnel: [w739 w741] -> w716
                          tunnel: [w737 w763] -> w733
                          tunnel: w732 -> [w739 w761]
                          tunnel: [FALSE w756] -> w718
                          tunnel: w726 -> [_ w755]
                          tunnel: [u16 0 ("Numeric") w754] -> w724
                          tunnel: [FALSE w743] -> w712
                          tunnel: w711 -> [_ w740]
                          frame False {
                          }
                          frame True {
                            n309 = flat-sequence {
                              tunnel: w761 -> [w772]
                              tunnel: [w776] -> w753
                              tunnel: [w774] -> w757
                              tunnel: w755 -> [w773]
                              tunnel: [w772] -> w762
                              tunnel: [w771] -> w754
                              frame #0 {
                                n310 = for {
                                tunnel: w773 -> [w789] mode=indexing
                                shift-right: [w784] -> w776
                                shift-left: u8[] [] -> [w783]
                                shift-right: [w781] -> w771
                                shift-left: u16 0 -> [w782]
                                i -> [w788]
                                n311 = Split Number(x=w789) -> (hi(x)=w780:u8, lo(x)=w779:u8)
                                n312 = Build Array(w780, w779) -> (w786:u8[])
                                n313 = Compound Arithmetic op=ADD(w782, w780, w779) -> (w781:u16)
                                n314 = Multiply(x=w788, y=2) -> (x*y=w785:i32)
                                n315 = Insert Into Array(array=w783, index=w785, new element=w786) -> (w784:u8[])
                                }
                                "CheckSum DataB" <- w771
                                n316 = Type Cast(type="", x=w771) -> (*(type *) &x=w774:string)
                              }
                            }
                            n317 = Byte Array To String(unsigned byte array=w753) -> (string=w742:string)
                            n318 = VISA Write(VISA resource name=w765, write buffer=w742, error in (no error)=w762) -> (VISA resource name out=w749:refnum<visa-resource-name>, error out=w748:errorcluster)  [unwired: 1 out]
                            n319 = flat-sequence {
                              tunnel: [w770] -> w746
                              tunnel: w748 -> [w769]
                              tunnel: [w769] -> w747
                              frame #0 {
                                n320 = call <vilib>:"High Resolution Relative Seconds.vi"() -> ("relative seconds"=w770:dbl)
                              }
                            }
                            n321 = while {
                              tunnel: w749 -> [w818]
                              tunnel: [w819] -> w766
                              tunnel: [w820] -> w750
                              tunnel: [w813] -> w760
                              tunnel: w747 -> [w809]
                              tunnel: w746 -> [w808]
                              tunnel: [w806] -> w744
                              stop <- w815 stop-if-true
                              n322 = VISA Read(VISA resource name=w818, byte count=u32 1, error in (no error)=w809) -> (VISA resource name out=w819:refnum<visa-resource-name>, read buffer=w813:string, return count=w814:u32, error out=w820:errorcluster)
                              n323 = call <vilib>:"High Resolution Relative Seconds.vi"() -> ("relative seconds"=w810:dbl)
                              n324 = Not Equal?(x=w814, y=u32 0) -> (x != y?=w816:bool)
                              n325 = property on="stop 6" class="Bool (strict)"() -> ("Value"=w807:bool)  [unwired: 2 in, 2 out]
                              n326 = Subtract(x=w810, y=w808) -> (x-y=w811:dbl)
                              n327 = Greater Or Equal?(x=w811, y=1.0) -> (x >= y?=w806:bool)
                              n328 = Compound Arithmetic op=OR(w816, w807, w806) -> (w815:bool)
                              n329 = property on="stop 6" class="Bool (strict)"("Value"=w806) -> ()  [unwired: 2 in, 2 out]
                            }
                            n330 = flat-sequence {
                              tunnel: w750 -> [w768]
                              tunnel: [w768] -> w751
                              tunnel: [w767] -> w752
                              frame #0 {
                                n331 = call <vilib>:"High Resolution Relative Seconds.vi"() -> ("relative seconds"=w767:dbl)
                              }
                            }
                            n332 = while {
                              tunnel: w766 -> [w804]
                              tunnel: [w801] -> w763
                              tunnel: w751 -> [w805]
                              tunnel: [w802] -> w764
                              tunnel: [w796] -> w759
                              tunnel: w752 -> [w792]
                              tunnel: [w790] -> w745
                              stop <- w797 stop-if-true
                              n333 = VISA Read(VISA resource name=w804, byte count=u32 1, error in (no error)=w805) -> (VISA resource name out=w801:refnum<visa-resource-name>, read buffer=w796:string, return count=w798:u32, error out=w802:errorcluster)
                              n334 = call <vilib>:"High Resolution Relative Seconds.vi"() -> ("relative seconds"=w795:dbl)
                              n335 = Not Equal?(x=w798, y=u32 0) -> (x != y?=w800:bool)
                              n336 = Subtract(x=w795, y=w792) -> (x-y=w794:dbl)
                              n337 = property on="stop 6" class="Bool (strict)"() -> ("Value"=w791:bool)  [unwired: 2 in, 2 out]
                              n338 = Greater Or Equal?(x=w794, y=1.0) -> (x >= y?=w790:bool)
                              n339 = Compound Arithmetic op=OR(w800, w791, w790) -> (w797:bool)
                              n340 = property on="stop 6" class="Bool (strict)"("Value"=w790) -> ()  [unwired: 2 in, 2 out]
                            }
                            n341 = Or(x=w745, y=w744) -> (x .or. y?=w743:bool)
                            n342 = Concatenate Strings(w759, w760) -> (w758:string)
                            n343 = call "Time Delay4"("error in (no error)"=w764, "Delay Time (s)"=w740) -> ("error out"=w741:errorcluster)  [unwired: 9 in]
                            n344 = Equal?(x=w757, y=w758) -> (x = y?=w756:bool)
                          }
                        }
                        n345 = property on="stop 6" class="Bool (strict)"("Value"=w712) -> ()  [unwired: 2 in, 2 out]
                        n346 = Build Array(w718) -> (w713:bool[])
                      }
                    }
                    frame True {
                      n347 = flat-sequence {
                        tunnel: w838 -> [w900]
                        tunnel: [w904] -> w831
                        tunnel: [w902] -> w832
                        tunnel: w839 -> [w901]
                        tunnel: [w900] -> w830
                        tunnel: [w899] -> w835
                        frame #0 {
                          n348 = for {
                            tunnel: w901 -> [w917] mode=indexing
                            shift-right: [w912] -> w904
                            shift-left: u8[] [] -> [w911]
                            shift-right: [w909] -> w899
                            shift-left: u16 0 -> [w910]
                            i -> [w916]
                            n349 = Split Number(x=w917) -> (hi(x)=w908:u8, lo(x)=w907:u8)
                            n350 = Build Array(w908, w907) -> (w914:u8[])
                            n351 = Compound Arithmetic op=ADD(w910, w908, w907) -> (w909:u16)
                            n352 = Multiply(x=w916, y=2) -> (x*y=w913:i32)
                            n353 = Insert Into Array(array=w911, index=w913, new element=w914) -> (w912:u8[])
                          }
                          "CheckSum Data" <- w899
                          n354 = Type Cast(type="", x=w899) -> (*(type *) &x=w902:string)
                        }
                      }
                      n355 = Build Array(w835) -> (w834:u16[])
                      n356 = Byte Array To String(unsigned byte array=w831) -> (string=w826:string)
                      n357 = VISA Write(VISA resource name=w829, write buffer=w826, error in (no error)=w830) -> (VISA resource name out=w828:refnum<visa-resource-name>, error out=w827:errorcluster)  [unwired: 1 out]
                      n358 = case shown="False" w833 {
                        tunnel: w828 -> [w857 w897]
                        tunnel: w827 -> [w850 w896]
                        tunnel: [w842 w896] -> w824
                        tunnel: [w855 w897] -> w840
                        tunnel: [w852 "\u0000\u0000"] -> w837
                        tunnel: [w843 FALSE] -> w823
                        tunnel: w822 -> [w841 _]
                        frame False {
                          n359 = flat-sequence {
                            tunnel: [w862] -> w851
                            tunnel: w850 -> [w861]
                            tunnel: [w861] -> w849
                            frame #0 {
                              n360 = call <vilib>:"High Resolution Relative Seconds.vi"() -> ("relative seconds"=w862:dbl)
                            }
                          }
                          n361 = while {
                            tunnel: w857 -> [w891]
                            tunnel: [w892] -> w858
                            tunnel: w849 -> [w890]
                            tunnel: [w893] -> w848
                            tunnel: [w885] -> w854
                            tunnel: w851 -> [w883]
                            tunnel: [w879] -> w844
                            stop <- w887 stop-if-true
                            n362 = VISA Read(VISA resource name=w891, byte count=u32 1, error in (no error)=w890) -> (VISA resource name out=w892:refnum<visa-resource-name>, read buffer=w885:string, return count=w886:u32, error out=w893:errorcluster)
                            n363 = call <vilib>:"High Resolution Relative Seconds.vi"() -> ("relative seconds"=w884:dbl)
                            n364 = Not Equal?(x=w886, y=u32 0) -> (x != y?=w888:bool)
                            n365 = Subtract(x=w884, y=w883) -> (x-y=w882:dbl)
                            n366 = property on="stop 6" class="Bool (strict)"() -> ("Value"=w880:bool)  [unwired: 2 in, 2 out]
                            n367 = Greater Or Equal?(x=w882, y=1.0) -> (x >= y?=w879:bool)
                            n368 = Compound Arithmetic op=OR(w888, w880, w879) -> (w887:bool)
                            n369 = property on="stop 6" class="Bool (strict)"("Value"=w879) -> ()  [unwired: 2 in, 2 out]
                          }
                          n370 = flat-sequence {
                            tunnel: w848 -> [w860]
                            tunnel: [w860] -> w847
                            tunnel: [w859] -> w846
                            frame #0 {
                              n371 = call <vilib>:"High Resolution Relative Seconds.vi"() -> ("relative seconds"=w859:dbl)
                            }
                          }
                          n372 = while {
                            tunnel: w858 -> [w877]
                            tunnel: [w874] -> w855
                            tunnel: w847 -> [w878]
                            tunnel: [w875] -> w856
                            tunnel: [w869] -> w853
                            tunnel: w846 -> [w865]
                            tunnel: [w863] -> w845
                            stop <- w870 stop-if-true
                            n373 = VISA Read(VISA resource name=w877, byte count=u32 1, error in (no error)=w878) -> (VISA resource name out=w874:refnum<visa-resource-name>, read buffer=w869:string, return count=w871:u32, error out=w875:errorcluster)
                            n374 = call <vilib>:"High Resolution Relative Seconds.vi"() -> ("relative seconds"=w866:dbl)
                            n375 = Not Equal?(x=w871, y=u32 0) -> (x != y?=w873:bool)
                            n376 = Subtract(x=w866, y=w865) -> (x-y=w867:dbl)
                            n377 = property on="stop 6" class="Bool (strict)"() -> ("Value"=w864:bool)  [unwired: 2 in, 2 out]
                            n378 = Greater Or Equal?(x=w867, y=1.0) -> (x >= y?=w863:bool)
                            n379 = Compound Arithmetic op=OR(w873, w864, w863) -> (w870:bool)
                            n380 = property on="stop 6" class="Bool (strict)"("Value"=w863) -> ()  [unwired: 2 in, 2 out]
                          }
                          n381 = Or(x=w845, y=w844) -> (x .or. y?=w843:bool)
                          n382 = Concatenate Strings(w853, w854) -> (w852:string)
                          n383 = call "Time Delay5"("error in (no error)"=w856, "Delay Time (s)"=w841) -> ("error out"=w842:errorcluster)  [unwired: 9 in]
                        }
                        frame True {
                        }
                      }
                      n384 = Equal?(x=w832, y=w837) -> (x = y?=w825:bool)
                      n385 = Build Array(w825) -> (w836:bool[])
                      n386 = property on="stop 6" class="Bool (strict)"("Value"=w823) -> ()  [unwired: 2 in, 2 out]
                    }
                  }
                  n387 = Not(x=w692) -> (.not. x?=w690:bool)
                }
                frame True {
                }
              }
            }
            "Array 3" <- w652
            "CheckSumArray" <- w648
          }
        }
        n388 = call <vilib>:"Clear Errors.vi"("error in (no error)"=w280) -> ("error out"=w279:errorcluster)  [unwired: 5 in, 1 out]
        n389 = property on="stop 6" class="Bool (strict)"(error in=w279) -> ("Value"=w234:bool)  [unwired: 1 in, 2 out]
        n390 = property on="Error List" class="Str"(error in=w279) -> (error out=w239:errorcluster, "Value"=w264:string)  [unwired: 1 in, 1 out]
        n391 = case shown="True" w271 {
          tunnel: ["" w420] -> w267
          tunnel: w234 -> [_ w417]
          tunnel: [TRUE ("Value") w417] -> w277
          tunnel: w239 -> [_ w416]
          frame False {
          }
          frame True {
            n392 = flat-sequence {
              tunnel: [w427] -> w419
              tunnel: [w421] -> w418
              tunnel: w416 -> [_]
              frame #0 {
                n393 = Format Date/Time String(time format string (%c)="%H:%M:%S ") -> (date/time string=w436:string)  [unwired: 2 in]
                n394 = Format Date/Time String(time format string (%c)="%H:%M:%S ") -> (date/time string=w435:string)  [unwired: 2 in]
                n395 = Format Date/Time String(time format string (%c)="%H:%M:%S ") -> (date/time string=w434:string)  [unwired: 2 in]
                n396 = Format Date/Time String(time format string (%c)="%H:%M:%S ") -> (date/time string=w433:string)  [unwired: 2 in]
                n397 = Concatenate Strings(w436, "Program failed !" ("string"), "\r\n") -> (w423:string)
                n398 = Concatenate Strings(w435, "Please check COM adaptor or try a different baudrate.") -> (w422:string)
                n399 = Concatenate Strings(w434, "Getting Driver version...", "\r\n") -> (w429:string)
                n400 = Concatenate Strings(w433, "Program success !" ("string")) -> (w428:string)
                n401 = Concatenate Strings(w423, w422) -> (w421:string)
                n402 = Concatenate Strings(w429, w428) -> (w427:string)
              }
            }
            n403 = Select(t=w418, s=w417, f=w419) -> (s? t:f=w420:string)
          }
        }
        n404 = Concatenate Strings(w267, "\r\n", w264) -> (w303:string)
        n405 = case shown="False" w234 {
          tunnel: w303 -> [w351 _]
          tunnel: [w350 w352] -> w286
          tunnel: w239 -> [w349 w352]
          frame False {
            n406 = property on="Error List" class="Str"(error in=w349, "Value"=w351) -> (error out=w350:errorcluster)  [unwired: 1 in, 1 out]
          }
          frame True {
          }
        }
        n407 = VISA Clear(VISA resource name=w299, error in (no error)=w286) -> (VISA resource name out=w287:refnum<visa-resource-name>, error out=w285:errorcluster)
        n408 = case shown="False" w234 {
          tunnel: w285 -> [w472 w519]
          tunnel: w287 -> [w471 _]
          tunnel: [w468 w519] -> w291
          tunnel: [w470 0 ("D Int out")] -> w297
          tunnel: [w469 FALSE] -> w296
          frame False {
            n409 = case shown="True" TRUE {
              tunnel: [w483 w488] -> w474
              tunnel: [w481 w487] -> w473
              tunnel: w472 -> [w482 w485]
              tunnel: w471 -> [w483 w484]
              frame False {
                n410 = call "Time Delay3"("error in (no error)"=w482) -> ("error out"=w481:errorcluster)  [unwired: 10 in]
              }
              frame True {
                w496 = u16 0 items=["None", "XON/XOFF", "RTS/CTS", "XON/XOFF & RTS/CTS", "DTR/DSR", "XON/XOFF & DTR/DSR"] ("flow control (0:none)")
                w495 = u16 10 items=["1.0"=10, "1.5"=15, "2.0"=20] ("stop bits (10: 1 bit)")
                w497 = T3 1073684533 items=["Service Request"=1073684491, "Trigger"=3221168138, "Clear"=1073684493, "VXI Signal"=1073684512, "VXI/VME Interrupt"=3221168161, "VXI/VME Sysfail"=1073684509, "VXI/VME Sysreset"=1073684510, "GPIB CIC"=1073684498, "GPIB Talk"=1073684499, "GPIB Listen"=1073684500, "PXI Interrupt"=1073684514, "Serial Break"=1073684515, "Serial TermChar"=1073684516, "Serial CTS"=1073684521, "Serial DSR"=1073684522, "Serial DCD"=1073684524, "Serial RI"=1073684526, "Serial Character"=1073684533, "USB Interrupt"=1073684535, "All Enabled"=1073709055] ("Event Type")
                n411 = call-poly "VISA Configure Serial Port"("VISA resource name"=w484, "timeout (10sec)"=u32 200, "Enable Termination\nChar (T)"=FALSE ("Enable Termination\nChar (T)"), "baud rate (9600)"=u32 230400, "data bits (8)"=u16 8, "parity (0:none)"=enum16{"None", "Odd", "Even", "Mark", "Space"}."None", "error in (no error)"=w485, "stop bits (10: 1 bit)"=w495, "flow control (0:none)"=w496) -> ("VISA resource name out"=w489:refnum<visa-resource-name>, "error out"=w490:errorcluster)  [unwired: 5 in]
                n412 = VISA Enable Event(8:w490, 10:w497, 11:w489) -> (0:w487:errorcluster, 3:w488:refnum<visa-resource-name>)  [unwired: 1 in]
              }
            }
            n413 = Byte Array To String(unsigned byte array=u8[] [73, 93, 62, 192, 16, 48, 0] ("output array")) -> (string=w478:string)
            n414 = VISA Write(VISA resource name=w474, write buffer=w478, error in (no error)=w473) -> (VISA resource name out=w480:refnum<visa-resource-name>, error out=w477:errorcluster)  [unwired: 1 out]
            n415 = flat-sequence {
              tunnel: w477 -> [w499]
              tunnel: [w499] -> w476
              tunnel: [w498] -> w475
              frame #0 {
                n416 = call <vilib>:"High Resolution Relative Seconds.vi"() -> ("relative seconds"=w498:dbl)
              }
            }
            n417 = while {
              tunnel: w476 -> [w516]
              tunnel: [w514] -> w468
              tunnel: w480 -> [w515]
              tunnel: w475 -> [w507]
              tunnel: [w502] -> w470
              tunnel: [w501] -> w469
              stop <- w504 stop-if-true
              n418 = call <vilib>:"High Resolution Relative Seconds.vi"() -> ("relative seconds"=w508:dbl)
              n419 = VISA Read(VISA resource name=w515, byte count=u32 11, error in (no error)=w516) -> (read buffer=w512:string, return count=w509:u32, error out=w514:errorcluster)  [unwired: 1 out]
              n420 = Subtract(x=w508, y=w507) -> (x-y=w505:dbl)
              n421 = String To Byte Array(string=w512) -> (unsigned byte array=w511:u8[])
              n422 = Not Equal To 0?(x=w509) -> (x != 0?=w501:bool)
              n423 = Greater Or Equal?(x=w505, y=3.0) -> (x >= y?=w503:bool)
              n424 = call "Data_Convert.vi"("Data Type"=u8 0, "Array"=w511) -> ("D Int out"=w502:i32)  [unwired: 2 out]
              n425 = property on="stop 6" class="Bool (strict)"() -> ("Value"=w500:bool)  [unwired: 2 in, 2 out]
              n426 = Compound Arithmetic op=OR(w500, w501, w503) -> (w504:bool)
            }
          }
          frame True {
          }
        }
        n427 = call <vilib>:"Clear Errors.vi"("error in (no error)"=w291) -> ("error out"=w288:errorcluster)  [unwired: 5 in, 1 out]
        n428 = property on="Error List" class="Str"(error in=w288) -> (error out=w238:errorcluster, "Value"=w265:string)  [unwired: 1 in, 1 out]
        n429 = case shown="False" w277 {
          tunnel: w297 -> [w406 _]
          tunnel: w296 -> [w405 _]
          tunnel: [w400 "" ("f")] -> w237
          tunnel: w238 -> [w402 _]
          frame False {
            n430 = flat-sequence {
              tunnel: w401 -> [w410]
              tunnel: [w409] -> _
              tunnel: w402 -> [_]
              tunnel: [w409] -> w400
              frame #0 {
                n431 = Format Date/Time String(time format string (%c)="%H:%M:%S ") -> (date/time string=w411:string)  [unwired: 2 in]
                n432 = Concatenate Strings(w411, w410) -> (w409:string)
              }
            }
            n433 = Format Into String(w406) -> (resulting string=w407:string)  [unwired: 3 in, 1 out]
            n434 = Concatenate Strings("Driver Version: " ("string"), w407) -> (w403:string)
            n435 = Select(t=w403, s=w405, f="Getting Driver version failed !") -> (s? t:f=w401:string)
          }
          frame True {
          }
        }
        n436 = Concatenate Strings(w237, "\r\n", w265) -> (w295:string)
        n437 = case shown="True" w234 {
          tunnel: [w347 w348] -> w298
          tunnel: w295 -> [w346 _]
          tunnel: w238 -> [w345 w348]
          frame False {
            n438 = property on="Error List" class="Str"(error in=w345, "Value"=w346) -> (error out=w347:errorcluster)  [unwired: 1 in, 1 out]
          }
          frame True {
          }
        }
        n439 = VISA Close(VISA resource name=w287, error in (no error)=w298) -> (error out=w273:errorcluster)
      }
    }
    n440 = for {
      tunnel: w87 -> [w151] mode=indexing
      shift-right: [w146] -> w85
      shift-left: u8[] [] -> [w145]
      shift-right: [w143] -> _
      shift-left: u16 0 -> [w144]
      i -> [w150]
      n441 = Split Number(x=w151) -> (hi(x)=w142:u8, lo(x)=w141:u8)
      n442 = Build Array(w142, w141) -> (w148:u8[])
      n443 = Compound Arithmetic op=ADD(w144, w142, w141) -> (w143:u16)
      n444 = Multiply(x=w150, y=2) -> (x*y=w147:i32)
      n445 = Insert Into Array(array=w145, index=w147, new element=w148) -> (w146:u8[])
    }
    "Full Text File" <- w85
    n446 = Array Size(array=w85) -> (size(s)=→"Size of Text File":i32)
    n447 = call <vilib>:"Clear Errors.vi"("error in (no error)"=w109) -> ("error out"=w98:errorcluster)  [unwired: 5 in, 1 out]
    n448 = property on="Next Button" class="Bool (strict)"(error in=w98, "Value"=w96, "Blinking"=w96) -> (error out=w108:errorcluster)  [unwired: 1 in, 1 out]
  }
  n449 = while {
    tunnel: w12 -> [_]
    i -> [w1058]
    stop <- FALSE stop-if-true
    (unwired) 1000
    n450 = event shown="[0] \"stop 7\": Value Change" {
      selector: _ -> [_ _]
      dyn-events: _ -> [_ _]
      timeout: _ -> [_ _]
      tunnel: w1058 -> [_ _]
      event "stop 7": Value Change {
        n451 = event-data() -> ()  [unwired: 1 in, 3 out]
        n452 = Two Button Dialog(message="Are you sure to close? ", 1:"No" ("F button name (\"Cancel\")"), 2:"Yes" ("T button name (\"OK\")")) -> (T button?=w1061:bool)
        n453 = property on="stop 6" class="Bool (strict)"("Value"=w1061) -> (error out=w1060:errorcluster)  [unwired: 2 in, 1 out]
        n454 = property on="stop 7" class="Bool (strict)"(error in=w1060, "Value"=w1061) -> (error out=w1062:errorcluster)  [unwired: 1 in, 1 out]
        n455 = case shown="True" w1061 {
          selector: w1061 -> [_ w1073]
          tunnel: w1062 -> [_ w1074]
          frame False {
          }
          frame True {
            w1071 = "\r\n"
            n456 = property on="Error List" class="Str"(error in=w1074) -> ("Value"=w1067:string)  [unwired: 1 in, 2 out]
            n457 = Format Date/Time String(time format string (%c)="%H:%M:%S") -> (date/time string=w1070:string)  [unwired: 2 in]
            n458 = Concatenate Strings(w1070, " Operation stopped by user") -> (w1066:string)
            n459 = Concatenate Strings(w1066, w1071, w1067, w1071) -> (w1075:string)
            n460 = property on="Error List" class="Str"("Value"=w1075) -> (error out=w1072:errorcluster)  [unwired: 2 in, 1 out]
            n461 = flat-sequence {
              tunnel: w1073 -> [_]
              tunnel: w1072 -> [_]
              frame #0 {
                n462 = property on="stop 7" class="Bool (strict)"("Value"=FALSE ("stop 7")) -> ()  [unwired: 2 in, 2 out]
              }
            }
          }
        }
      }
      event Timeout {
        n463 = event-data() -> ()  [unwired: 1 in, 3 out]
        n464 = disable-structure shown="Disabled" {
          frame Disabled {
            n465 = property on="Error List" class="Str" props=["Text", "Scroll Position"]() -> ()  [unwired: 3 in, 2 out]
          }
          frame Enabled {
          }
        }
      }
    }
  }
  n466 = disable-structure shown="Disabled" {
    frame Disabled {
      n467 = call <vilib>:"Application Directory.vi"() -> ("Application Directory"=w1081:path)
      n468 = Build Path(base path=w1081, name or relative path="ans.txt") -> (appended path=w1080:path)
      n469 = Open/Create/Replace File(file path (use dialog)=w1080, operation (0:open)=T4."open or create") -> (refnum out=w1077:refnum<file>, error out=w1078:errorcluster)  [unwired: 4 in, 1 out]
      n470 = for {
        tunnel: _ -> [w1093] mode=indexing
        tunnel: w1078 -> [w1091]
        tunnel: w1077 -> [w1090]
        i -> [w1086]
        n471 = Quotient & Remainder(x=w1086, y=24 ("x")) -> (x-y*floor(x/y)=w1084:i32)  [unwired: 1 out]
        n472 = Format Into String(format string="%02x", w1093) -> (resulting string=w1089:string)  [unwired: 2 in, 1 out]
        n473 = Equal?(x=w1084, y=0) -> (x = y?=w1087:bool)
        n474 = case shown="True" w1087 {
          tunnel: w1089 -> [w1096 w1099]
          tunnel: [w1095 w1098] -> w1088
          frame False {
            n475 = call <vilib>:"Space Constant.vi"() -> ("String"=w1094:string)
            n476 = Concatenate Strings(w1096, w1094) -> (w1095:string)
          }
          frame True {
            n477 = Concatenate Strings(w1099, "\r\n") -> (w1098:string)
          }
        }
        n478 = Write to Text File(file (use dialog)=w1090, text=w1088, error in=w1091) -> ()  [unwired: 1 in, 3 out]
      }
    }
    frame Enabled {
    }
  }
  n479 = disable-structure shown="Enabled" {
    disable-tunnel: _ -> [w1103 _]
    disable-tunnel: w31 -> [w1102 w1104]
    disable-tunnel: [w1101 w1104] -> w30
    frame Disabled {
      n480 = call <vilib>:"Close Config Data.vi"("error in (no error)"=w1102, "write file if changed (T)"=TRUE, "refnum"=w1103) -> ("error out"=w1101:errorcluster)  [unwired: 8 out]
    }
    frame Enabled {
    }
  }
  "error out" <- w30
